vi "FindInstruments.vi"(8 "error in (no error)":errorcluster, 11 "KIM101 in":refnum<class "KIM101.lvclass">) -> (0 "error out":errorcluster, 3 "KIM101 out":refnum<class "KIM101.lvclass">)   [LabVIEW 2023, in "KIM101.lvlib" / "KIM101.lvclass"]
uses:
  KIM101.lvclass
  KIM101.lvclass/KIM101.ctl
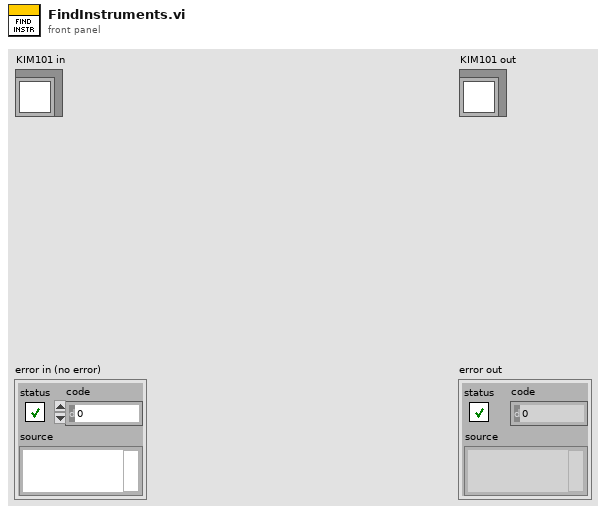
[diagram p1: front panel]
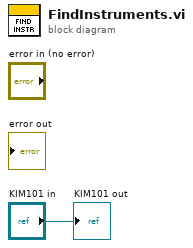
[diagram p0: block diagram]
diagram:
  "KIM101 out" <- "KIM101 in"
